vi "McP789A-3-Global-Info.vi"() -> ()   [LabVIEW 2024]
panel:
  in  "PixDist(mm)":dbl
  in  "FocalLength":dbl
  in  "MirrorAngle":dbl
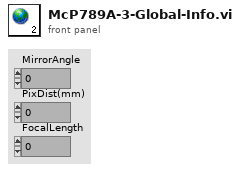
[diagram p1: front panel]
diagram:
